vi "Heat Equation Solver(lv_gpu).vi"() -> ()   [LabVIEW 2020]
doc: "Solves the heat equation in a two-dimensional area using a Finite Element Method."
uses:
  <vilib>/Utility/miscctls.llb/LVPointDoubleTypeDef.ctl
  <vilib>/picture/3D Picture Control/Object/Create Object (name).vi
  <vilib>/addons/lvgpu/lvcuda/CUDA SGL Device Ptr/Download 2D Data.vi
  <vilib>/addons/lvgpu/lvcuda/CUDA SGL Device Ptr/Download 1D Data.vi
  <vilib>/addons/lvgpu/lvcublas/SGEMM (aAB+bC).vi
  <vilib>/addons/lvgpu/lvcuda/CUDA SGL Device Ptr/Upload 1D Data.vi
  <vilib>/addons/lvgpu/lvcuda.lvlib
  <vilib>/addons/lvgpu/lvcublas.lvlib
  subVIs/Heat Equation Solver.lvlib
  <vilib>/addons/lvgpu/lvcuda/CUDA SGL Device Ptr/CUDA SGL Device Ptr.lvclass
  <vilib>/picture/3D Picture Control/NI_3D Picture Control.lvlib
  <vilib>/ptbypt/NI_PtbyPt.lvlib
panel:
  out "stop display":bool
  out "Heat Map":sgl[](array[numeric])
  out "time graph":dbl(graph)
  out "Device Name":string
  out "Error Status":errorcluster
  out "CUDA Version":string
  in  "Device ID":i32 min=0 max=0
  in  "radius":dbl(slide)=0.15 caption="Radius" min=0.1 max=0.3 step=0.01 scale=0.1..0.2
  out "sol":refnum<vi>(3d-picture) caption="Heat Distribution"
  out "colorbar":sgl[][](graph)
  out "tri":cluster{"X":dbl[], "Y":dbl[]}[](graph) caption="Triangulation"
  out "time":dbl[unit] format="%#_4p"
  in  "stop":bool
  # "Heat Equation Solver based on NI's GPU Toolkit"
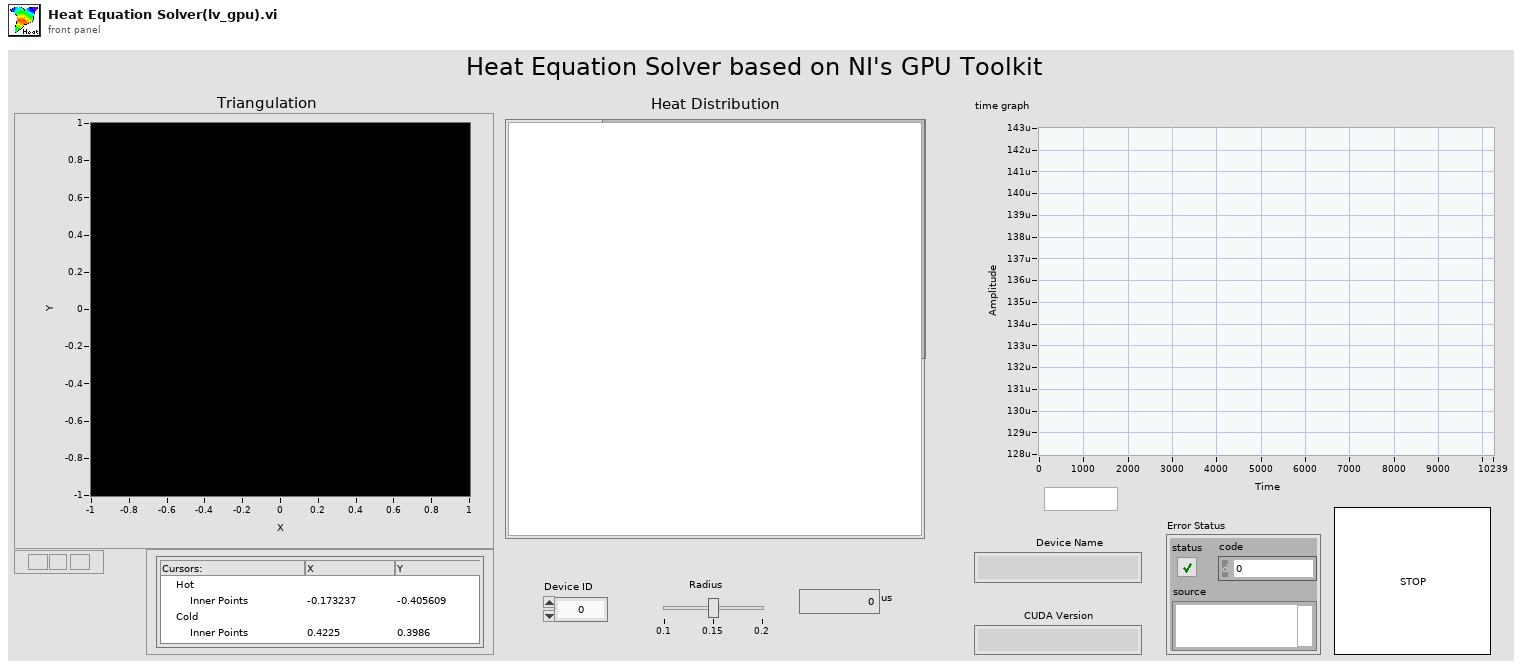
[diagram p1: front panel]
types:
  T1 = typedef "Heat Equation Solver.lvlib/FEM Grid.ctl" = cluster{"X":dbl[], "Y":dbl[], "Trianglation":i32[][]}
  T2 = typedef "NI_Matrix.lvlib/RealMatrix.ctl" = dbl[][]
  T3 = typedef "LVPointDoubleTypeDef.ctl" = cluster{"X":dbl, "Y":dbl}
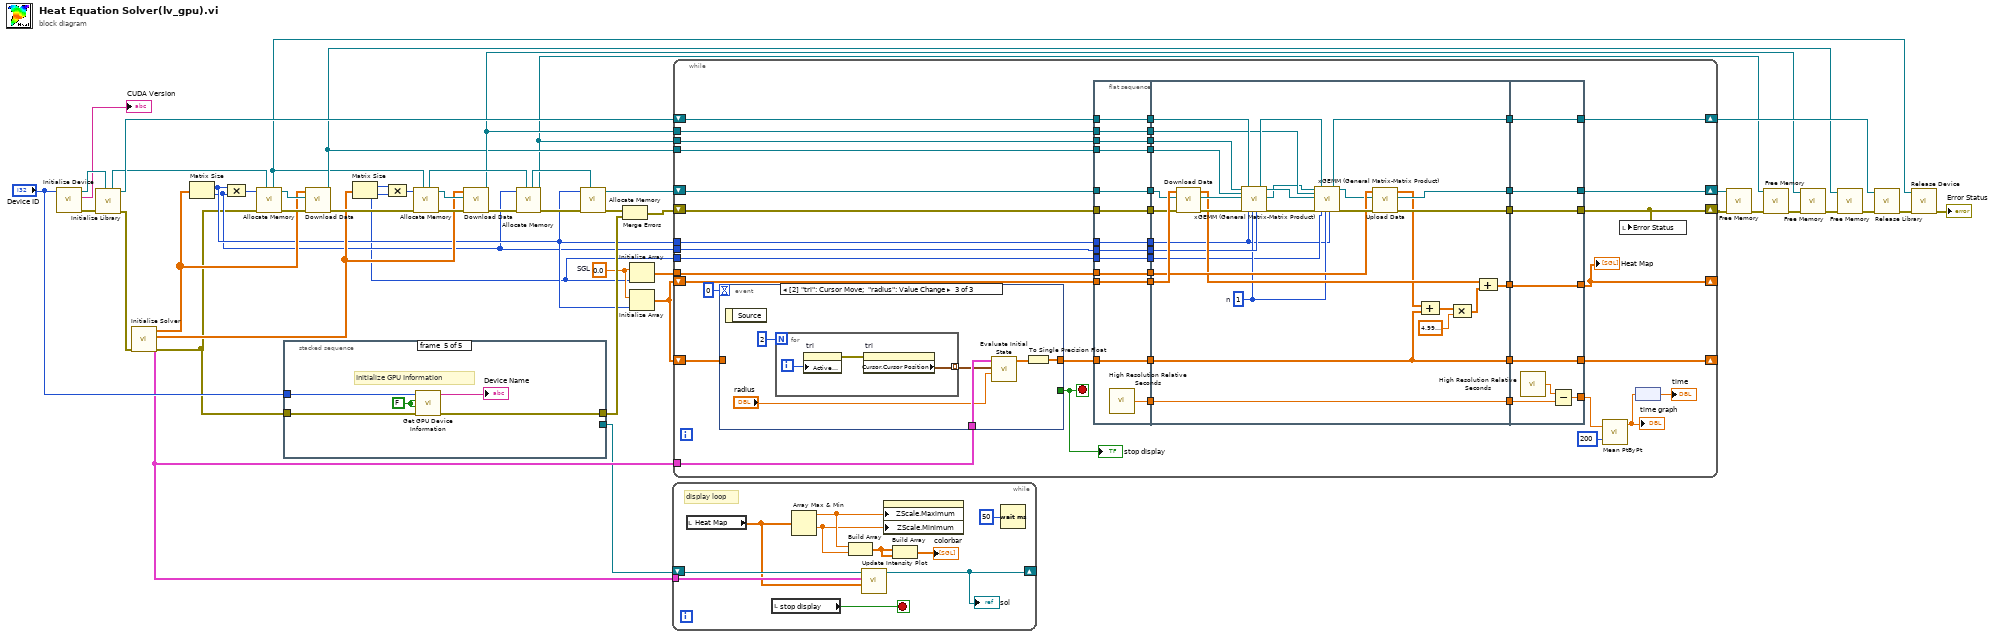
[diagram p0: block diagram]
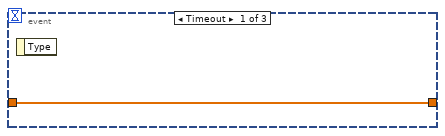
[diagram p2: hidden frame]
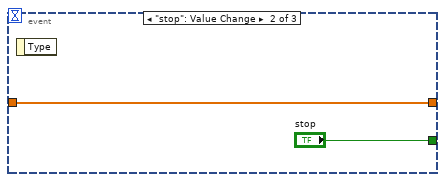
[diagram p3: hidden frame]
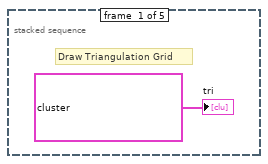
[diagram p4: hidden frame]
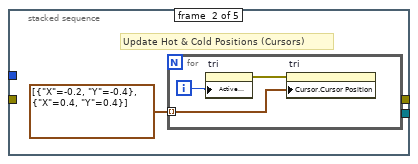
[diagram p5: hidden frame]
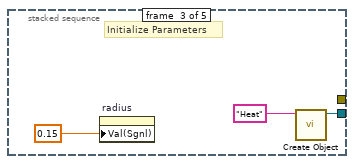
[diagram p6: hidden frame]
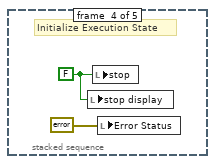
[diagram p7: hidden frame]
diagram:
  w13 = sgl 0.0  # SGL
  n1 = call <vilib>:"Initialize Device.vi"("CUDA Device ID"="Device ID") -> ("error out"=w42:errorcluster, "CUDA Version"=→"CUDA Version":string, "CUDA Context"=w44:refnum<class "CUDA Context.lvclass">)  [unwired: 8 in]
  n2 = call <vilib>:"Initialize Library.vi"("CUDA Context in"=w44, "error in"=w42) -> ("error out"=w22:errorcluster, "CUBLAS Handle"=w46:refnum<class "CUBLAS Handle.lvclass">, "CUDA Context out"=w41:refnum<class "CUDA Context.lvclass">)  [unwired: 6 in, 1 out]
  n3 = call "Initialize Solver.vi"("error in"=w22) -> ("error out"=w5:errorcluster, "FEM Grid"=w2:T1, "Mass"=w23:T2, "Stiffness"=w24:T2)  [unwired: 7 in]
  n4 = Matrix Size(0:w24) -> (1:w9:i32, 2:w8:i32)
  n5 = Compound Arithmetic op=MULTIPLY(w9, w8) -> (w30:i32)
  n6 = call-poly <vilib>:"Allocate Memory.vi"("CUDA Context in"=w41, "error in"=w5, "size in elements"=w30) -> ("error out"=w28:errorcluster, "CUDA SGL Device Ptr out"=w38:refnum<class "CUDA SGL Device Ptr.lvclass">, "CUDA Context out"=w15:refnum<class "CUDA Context.lvclass">)  [unwired: 6 in]
  n7 = stacked-sequence {
    tunnel: [_ _ w54 _ _] -> w1
    tunnel: "Device ID" -> [_ _ _ _ w62]
    tunnel: w5 -> [_ _ _ _ w60]
    tunnel: [_ _ _ _ w59] -> w47
    frame #0 {
      # "Draw Triangulation Grid"
      "tri" <- cluster{"X":dbl[], "Y":dbl[]}[] [{"X"=array[689 elements], "Y"=array[689 elements]}, {"X"=[-0.825, -0.8029029130879204, -0.8, -0.775, -0.7625, -0.7375, -0.725, -0.7, -0.6875, -0.6625, -0.65, -0.625, -0.6125, -0.5875, -0.575, -0.55, -0.5375, -0.5125, -0.5, -0.475, -0.4625, -0.44999999999999996, -0.44999999999999996, -0.44999999999999996, -0.44999999999999996, -0.44999999999999996, -0.44375, -0.44375, -0.44375, -0.4375, -0.4375, -0.43125, -0.43125, -0.42500000000000004, -0.42500000000000004, -0.42500000000000004, -0.41250000000000003, -0.4125, -0.4, -0.3875, -0.3875, -0.38125, -0.375, -0.375, -0.36875, -0.36250000000000004, -0.35625, -0.35, -0.35, -0.35, -0.34375, -0.34375, -0.3375, -0.3375, -0.3375, -0.33749999999999997, -0.33125, -0.32499999999999996, -0.32499999999999996, -0.32499999999999996, -0.3125, -0.3125, -0.2875, -0.275, -0.26249999999999996, -0.2375, -0.23124999999999996, -0.19999999999999996, -0.19999999999999996, -0.16874999999999996, -0.16249999999999998, -0.13749999999999996, -0.125, -0.09999999999999998, -0.08750000000000002, -0.0625, -0.050000000000000044, -0.025000000000000022, -0.012500000000000067, 0.012499999999999956, 0.02499999999999991, 0.025000000000000022, 0.03750000000000009, 0.03750000000000009, 0.03750000000000009, 0.03750000000000009, 0.03750000000000009, 0.0625, 0.10000000000000009, 0.10000000000000009, 0.13750000000000007, 0.13750000000000007, 0.17500000000000004, 0.17500000000000004, 0.19374999999999998, 0.2124999999999999, 0.21250000000000002, 0.2437499999999999, 0.25, 0.2749999999999999, 0.2875, 0.32499999999999996, 0.3374999999999999, 0.36249999999999993, 0.375, 0.3999999999999999, 0.4125000000000001, 0.4375, 0.45000000000000007, 0.4750000000000001, 0.48750000000000004, 0.5125000000000001, 0.525, 0.55, 0.5625, 0.5875, 0.6, 0.625, 0.6375, 0.65625, 0.6625000000000001, 0.6625000000000001, 0.6625000000000001, 0.6687500000000001, 0.6749999999999999, 0.675, 0.675, 0.675, 0.675, 0.68125, 0.6875, 0.6875, 0.7, 0.7124999999999999, 0.7124999999999999, 0.725, 0.7375, 0.75, 0.7625000000000001, 0.7875000000000001, 0.7875000000000001, 0.80625, 0.825, 0.8250000000000001, 0.85625, 0.8625, 0.8875, 0.9, 0.90625, 0.9249999999999999, 0.9375, 0.9624999999999999], "Y"=[0.575, 0.5529029130879203, 0.6000000000000001, 0.5249999999999999, 0.61875, 0.5125, 0.6375, 0.5, 0.65625, 0.475, 0.675, 0.44999999999999996, 0.69375, 0.42499999999999993, 0.7124999999999999, 0.3999999999999999, 0.71875, 0.36249999999999993, 0.7250000000000001, 0.32499999999999996, 0.7312500000000001, -0.7875, -0.75, -0.7125, -0.675, -0.6375, -0.825, -0.6, 0.2875, -0.8625, -0.5625, -0.9, -0.525, -0.9375, -0.48750000000000004, 0.7375, -0.45, 0.25, -0.4125, -0.375, 0.74375, 0.21875, -0.925, -0.3375, -0.3, -0.26249999999999996, -0.22499999999999998, -0.1875, 0.1875, 0.75, -0.8875, -0.15000000000000002, -0.11250000000000004, -0.07500000000000001, -0.03749999999999998, 0.15000000000000002, 5.551115123125783e-17, 0.03750000000000009, 0.07500000000000007, 0.11250000000000004, -0.85, 0.75, -0.8125, 0.75, -0.775, 0.75, -0.74375, -0.7125, 0.75, -0.68125, 0.74375, -0.65, 0.7375, -0.61875, 0.71875, -0.5875, 0.7, -0.55625, 0.6749999999999999, -0.525, 0.6499999999999999, -0.4875, -0.44999999999999996, -0.4125, -0.375, -0.3375, -0.30000000000000004, 0.6124999999999999, -0.32499999999999996, 0.575, -0.35, 0.54375, -0.375, 0.5125, 0.5499999999999999, 0.5874999999999999, -0.36875, 0.625, -0.36250000000000004, 0.6625000000000001, -0.35000000000000003, -0.3375, 0.7, -0.31875000000000003, 0.7062499999999999, -0.30000000000000004, 0.7124999999999999, -0.28125, 0.725, -0.26249999999999996, 0.7375, -0.24374999999999997, 0.7375, -0.22499999999999998, 0.7375, -0.20625, 0.74375, -0.1875, 0.75, -0.16249999999999998, 0.08749999999999991, 0.13124999999999998, 0.17500000000000004, 0.04999999999999993, 0.75, -0.0625, -0.025000000000000022, 0.012499999999999956, 0.21250000000000002, -0.09999999999999998, -0.13749999999999996, 0.25, 0.2875, 0.32499999999999996, 0.75, 0.36249999999999993, 0.3999999999999999, 0.75, 0.4375, 0.4750000000000001, 0.75, 0.5125000000000001, 0.55, 0.75, 0.5875, 0.75, 0.625, 0.75, 0.64375, 0.6625, 0.75, 0.7]}, {"X"=array[456 elements], "Y"=array[456 elements]}, {"X"=array[7640 elements], "Y"=array[7640 elements]}] ("Triangulation Plot")
    }
    frame #1 {
      # "Update Hot & Cold Positions (Cursors)"
      n8 = for {
        tunnel: T3[] [{"X"=-0.2, "Y"=-0.4}, {"X"=0.4, "Y"=0.4}] -> [w51] mode=indexing
        i -> [w52]
        n9 = property on="tri" class="XYGraph (strict)"("Active Cursor"=w52) -> (error out=w50:errorcluster)  [unwired: 2 in, 1 out]
        n10 = property on="tri" class="XYGraph (strict)"(error in=w50, "Cursor.Cursor Position"=w51) -> ()  [unwired: 1 in, 2 out]
      }
    }
    frame #2 {
      # "Initialize Parameters"
      n11 = property on="radius" class="Slide (strict)"("Val(Sgnl)"=0.15 ("r")) -> ()  [unwired: 2 in, 2 out]
      n12 = call-poly <vilib>:"Create Object.vi"("Name"="Heat") -> ("Scene:New Object"=w54:refnum<vi>)  [unwired: 9 in, 1 out]
    }
    frame #3 {
      w56 = FALSE ("stop")
      # "Initialize Execution State"
      n13 = local write "stop display"(w56) -> ()
      n14 = local write "stop"(w56) -> ()
      n15 = local write "Error Status"(errorcluster {"status"=FALSE, "code"=0, "source"=""} ("Error Status")) -> ()
    }
    frame #4 {
      w58 = FALSE ("Test Device Execution?")
      # "Initialize GPU Information"
      n16 = call "Get GPU Device Information.vi"("error in"=w60, "Reset Device?"=w58, "Test Device Execution?"=w58, "Device ID"=w62) -> ("error out"=w59:errorcluster, "Device Name"=→"Device Name":string)  [unwired: 1 in, 5 out]
    }
  }
  n17 = call-poly <vilib>:"Download Data.vi"("error in"=w28, "dst in"=w38, "src in"=w24) -> ("error out"=w27:errorcluster, "dst out"=w18:refnum<class "CUDA SGL Device Ptr.lvclass">)  [unwired: 6 in, 1 out]
  n18 = Matrix Size(0:w23) -> (1:w7:i32, 2:w29:i32)
  n19 = Compound Arithmetic op=MULTIPLY(w7, w29) -> (w39:i32)
  n20 = call-poly <vilib>:"Allocate Memory.vi"("CUDA Context in"=w15, "error in"=w27, "size in elements"=w39) -> ("error out"=w26:errorcluster, "CUDA SGL Device Ptr out"=w37:refnum<class "CUDA SGL Device Ptr.lvclass">, "CUDA Context out"=w40:refnum<class "CUDA Context.lvclass">)  [unwired: 6 in]
  n21 = call-poly <vilib>:"Download Data.vi"("error in"=w26, "dst in"=w37, "src in"=w23) -> ("error out"=w25:errorcluster, "dst out"=w19:refnum<class "CUDA SGL Device Ptr.lvclass">)  [unwired: 6 in, 1 out]
  n22 = call-poly <vilib>:"Allocate Memory.vi"("CUDA Context in"=w40, "error in"=w25, "size in elements"=w8) -> ("error out"=w14:errorcluster, "CUDA SGL Device Ptr out"=w11:refnum<class "CUDA SGL Device Ptr.lvclass">, "CUDA Context out"=w21:refnum<class "CUDA Context.lvclass">)  [unwired: 6 in]
  n23 = call-poly <vilib>:"Allocate Memory.vi"("CUDA Context in"=w21, "error in"=w14, "size in elements"=w9) -> ("error out"=w4:errorcluster, "CUDA SGL Device Ptr out"=w20:refnum<class "CUDA SGL Device Ptr.lvclass">)  [unwired: 6 in, 1 out]
  n24 = Merge Errors(w4, w47) -> (w3:errorcluster)
  n25 = Initialize Array(w13, w7) -> (w12:sgl[])
  n26 = Initialize Array(w13, w9) -> (w45:sgl[])
  n27 = while {
    tunnel: w2 -> [w71]
    shift-right: [w65] -> _
    shift-left: w1 -> [w72]
    stop <- w68 stop-if-true
    # "display loop"
    n28 = local read "Heat Map"() -> (w67:sgl[])
    n29 = local read "stop display"() -> (w68:bool)
    n30 = Array Max & Min(array=w67) -> (max value=w64:sgl, min value=w63:sgl)  [unwired: 2 out]
    n31 = Build Array(w64, w63) -> (w69:sgl[])
    n32 = call "Update Intensity Plot.vi"("Z"=w67, "FEM Grid"=w71, "FEM plot in"=w72) -> ("FEM plot out"=w65:refnum<vi>)  [unwired: 8 in]
    "sol" <- w65
    n33 = property on="colorbar" class="IntGraph (strict)"("ZScale.Maximum"=w64, "ZScale.Minimum"=w63) -> ()  [unwired: 2 in, 2 out]
    n34 = Build Array(w69, w69) -> (→"colorbar":sgl[][])
    n35 = Wait (ms)(milliseconds to wait=u32 50) -> ()  [unwired: 1 out]
  }
  n36 = while {
    tunnel: w2 -> [w100]
    shift-right: [w101] -> _
    shift-left: w45 -> [w104]
    shift-right: [w106] -> _
    shift-left: w45 -> [w107]
    shift-right: [w85] -> w36
    shift-left: w46 -> [w98]
    shift-right: [w87] -> w17
    shift-left: w20 -> [w94]
    shift-right: [w86] -> w16
    shift-left: w3 -> [w92]
    tunnel: w19 -> [w103]
    tunnel: w18 -> [w102]
    tunnel: w11 -> [w96]
    tunnel: w9 -> [w82]
    tunnel: w12 -> [w90]
    tunnel: w8 -> [w80]
    tunnel: w7 -> [w78]
    stop <- w109 stop-if-true
    n37 = event shown="[2] \"tri\": Cursor Move;  \"radius\": Value Change" {
      selector: _ -> [_ _ _]
      dyn-events: _ -> [_ _ _]
      timeout: 0 -> [_ _ _]
      tunnel: [w169 w170 w172] -> w73
      tunnel: [_ "stop" _] -> w109
      tunnel: w100 -> [_ _ w177]
      tunnel: w107 -> [w169 w170 _]
      event Timeout {
        n38 = event-data() -> ()  [unwired: 1 in, 1 out]
      }
      event "stop": Value Change {
        n39 = event-data() -> ()  [unwired: 1 in, 1 out]
      }
      event "tri": Cursor Move; "radius": Value Change {
        n40 = event-data() -> ()  [unwired: 1 in, 1 out]
        n41 = for {
          N: 2 -> [_]
          tunnel: [w178] -> w175 mode=indexing
          i -> [w180]
          n42 = property on="tri" class="XYGraph (strict)"("Active Cursor"=w180) -> (error out=w179:errorcluster)  [unwired: 2 in, 1 out]
          n43 = property on="tri" class="XYGraph (strict)"(error in=w179) -> ("Cursor.Cursor Position"=w178:T3)  [unwired: 1 in, 2 out]
        }
        n44 = call "Evaluate Initial State.vi"("r"="radius", "Heat Source"=w175, "FEM Grid"=w177) -> ("Initial"=w173:dbl[])  [unwired: 8 in]
        n45 = To Single Precision Float(number=w173) -> (single precision float=w172:sgl[])
      }
    }
    "stop display" <- w109
    n46 = flat-sequence {
      tunnel: w103 -> [w128]
      tunnel: w102 -> [w129]
      tunnel: [w129] -> w116
      tunnel: [w128] -> w115
      tunnel: [w126] -> w114
      tunnel: [w127] -> w113
      tunnel: w104 -> [w126]
      tunnel: w73 -> [w125]
      tunnel: [w125] -> w108
      tunnel: [w124] -> w99
      tunnel: w98 -> [w124]
      tunnel: [w123] -> w97
      tunnel: w96 -> [w123]
      tunnel: [w122] -> w95
      tunnel: w94 -> [w122]
      tunnel: [w121] -> w93
      tunnel: w92 -> [w121]
      tunnel: [w120] -> w91
      tunnel: w90 -> [w120]
      tunnel: [w119] -> w83
      tunnel: w82 -> [w119]
      tunnel: [w118] -> w81
      tunnel: w80 -> [w118]
      tunnel: [w117] -> w79
      tunnel: w78 -> [w117]
      tunnel: [w160] -> w112
      tunnel: w116 -> [w156]
      tunnel: w115 -> [w152]
      tunnel: w114 -> [w150]
      tunnel: w113 -> [w159]
      tunnel: [w159] -> w111
      tunnel: w108 -> [w157]
      tunnel: [w157] -> w105
      tunnel: w99 -> [w155]
      tunnel: w97 -> [w147]
      tunnel: w95 -> [w148]
      tunnel: w93 -> [w146]
      tunnel: w91 -> [w142]
      tunnel: [w140] -> w89
      tunnel: [w139] -> w88
      tunnel: [w135] -> w84
      tunnel: w83 -> [w130]
      tunnel: w81 -> [w133]
      tunnel: w79 -> [w131]
      tunnel: [w168] -> w101
      tunnel: w112 -> [w168]
      tunnel: w111 -> [w167]
      tunnel: [w166] -> w106
      tunnel: w105 -> [w166]
      tunnel: w89 -> [w163]
      tunnel: [w164] -> w87
      tunnel: w88 -> [w164]
      tunnel: [w163] -> w86
      tunnel: [w162] -> w85
      tunnel: w84 -> [w162]
      tunnel: [w161] -> w76
      frame #0 {
        n47 = call <vilib>:"High Resolution Relative Seconds.vi"() -> ("relative seconds"=w127:dbl)
      }
      frame #1 {
        w132 = 1  # n
        n48 = call-poly <vilib>:"Download Data.vi"("error in"=w146, "dst in"=w148, "src in"=w150) -> ("error out"=w151:errorcluster, "dst out"=w149:refnum<class "CUDA SGL Device Ptr.lvclass">, "src out"=w137:sgl[])  [unwired: 6 in]
        n49 = call-poly <vilib>:"xGEMM (General Matrix-Matrix Product).vi"("C"=w147, "A in"=w156, "B in"=w149, "error in"=w151, "CUBLAS Handle in"=w155, "m"=w130, "n"=w132, "k"=w133) -> ("CUBLAS Handle out"=w153:refnum<class "CUBLAS Handle.lvclass">, "aAB+bC"=w154:refnum<class "CUDA SGL Device Ptr.lvclass">, "B out"=w144:refnum<class "CUDA SGL Device Ptr.lvclass">, "error out"=w145:errorcluster)  [unwired: 7 in, 1 out]
        n50 = call-poly <vilib>:"xGEMM (General Matrix-Matrix Product).vi"("C"=w144, "A in"=w152, "B in"=w154, "error in"=w145, "CUBLAS Handle in"=w153, "m"=w131, "n"=w132, "k"=w130) -> ("CUBLAS Handle out"=w135:refnum<class "CUBLAS Handle.lvclass">, "aAB+bC"=w141:refnum<class "CUDA SGL Device Ptr.lvclass">, "error out"=w143:errorcluster)  [unwired: 7 in, 2 out]
        n51 = call-poly <vilib>:"Upload Data.vi"("error in"=w143, "src in"=w141, "dst in"=w142) -> ("error out"=w140:errorcluster, "src out"=w139:refnum<class "CUDA SGL Device Ptr.lvclass">, "dst out"=w134:sgl[])  [unwired: 6 in]
        n52 = Compound Arithmetic op=ADD(w134, w157) -> (w158:sgl[])
        n53 = Compound Arithmetic op=MULTIPLY(w158, sgl 5e-05 ("dt")) -> (w136:sgl[])
        n54 = Compound Arithmetic op=ADD(w137, w136) -> (w160:sgl[])
      }
      frame #2 {
        n55 = call <vilib>:"High Resolution Relative Seconds.vi"() -> ("relative seconds"=w165:dbl)
        n56 = Subtract(x=w165, y=w167) -> (x-y=w161:dbl)
      }
    }
    n57 = call <vilib>:"Mean PtByPt.vi"("x"=w76, "sample length"=200) -> ("mean"=w75:dbl)  [unwired: 2 in, 1 out]
    "time graph" <- w75
    n58 = local write "Error Status"(w86) -> ()
    n59 = node(w75) -> (→"time":dbl[unit])
    "Heat Map" <- w101
  }
  n60 = call-poly <vilib>:"Free Memory.vi"("error in"=w16, "CUDA SGL Device Ptr in"=w17) -> ("error out"=w31:errorcluster)  [unwired: 9 in]
  n61 = call-poly <vilib>:"Free Memory.vi"("error in"=w31, "CUDA SGL Device Ptr in"=w11) -> ("error out"=w32:errorcluster)  [unwired: 9 in]
  n62 = call-poly <vilib>:"Free Memory.vi"("error in"=w32, "CUDA SGL Device Ptr in"=w19) -> ("error out"=w33:errorcluster)  [unwired: 9 in]
  n63 = call-poly <vilib>:"Free Memory.vi"("error in"=w33, "CUDA SGL Device Ptr in"=w18) -> ("error out"=w34:errorcluster)  [unwired: 9 in]
  n64 = call <vilib>:"Release Library.vi"("error in"=w34, "CUBLAS Handle"=w36) -> ("error out"=w35:errorcluster)  [unwired: 9 in]
  n65 = call <vilib>:"Release Device.vi"("error in"=w35, "CUDA Context in"=w15) -> ("error out"=→"Error Status":errorcluster)  [unwired: 9 in]
